vi "Pop First Streaming Buffer.vi"(8 "error in (no error)":errorcluster, 9 "Timeout (ms) Default: -1":i32=-1, 10 "Buffer in":refnum<class "Buffer.lvclass">, 11 "Camera in":refnum<class "Camera.lvclass">) -> (0 "error out":errorcluster, 2 "Buffer":refnum<class "Buffer.lvclass">, 3 "Camera":refnum<class "Camera.lvclass">)   [LabVIEW 2020, in "Camera.lvclass"]
uses:
  Camera.lvclass
  Buffer/Buffer.lvclass
  Camera.lvclass/Camera.ctl
  Buffer/Buffer.lvclass/Buffer.ctl
  bin/gindustrialcam_32-1.dll
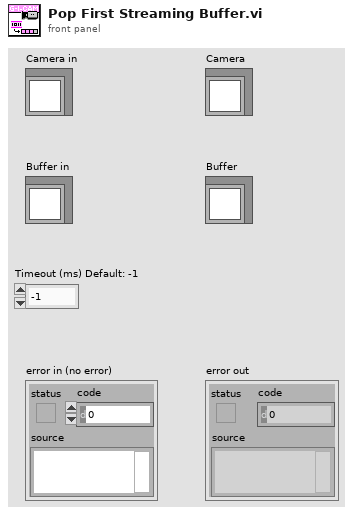
[diagram p1: front panel]
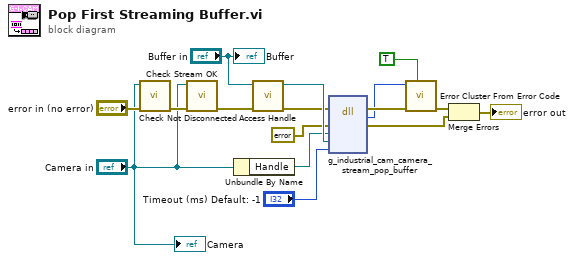
[diagram p0: block diagram]
diagram:
  n1 = call "Check Not Disconnected.vi"("error in (no error)"="error in (no error)", "Camera in"="Camera in") -> ("error out"=w12:errorcluster)  [unwired: 9 in]
  n2 = call "Check Stream OK.vi"("error in (no error)"=w12, "Camera in"="Camera in") -> ("error out"=w10:errorcluster)  [unwired: 9 in]
  n3 = Unbundle By Name("Camera in") -> ("Handle"=w8:refnum<data-value>)
  n4 = call "Access Handle.vi"("error in (no error)"=w10, "Buffer"="Buffer in") -> ("error out"=w15:errorcluster, "Handle"=w16:refnum<data-value>)  [unwired: 8 in]
  n5 = dll-call lib="C:/Workspace/SSDC/g-industrial-camera/LabVIEW/g_industrial_cam/bin/gindustrialcam_*-1.*" fn="g_industrial_cam_camera_stream_pop_buffer"(error in=w15, "err"=errorcluster {"status"=FALSE, "code"=0, "source"=""} ("error constant"), "cam_edvr"=w8, "buffer_edvr"=w16, "timeout_ms"="Timeout (ms) Default: -1") -> (error out=w7:errorcluster, "Mg_Error"=w6:i32, "err"=w2:errorcluster)  [unwired: 5 in, 1 out]
  n6 = call <vilib>:"Error Cluster From Error Code.vi"("show call chain? (False)"=TRUE, "error in (no error)"=w7, "error code (0)"=w6) -> ("error out"=w5:errorcluster)  [unwired: 6 in]
  n7 = Merge Errors(w5, w2) -> (→"error out":errorcluster)
  "Camera" <- "Camera in"
  "Buffer" <- "Buffer in"
